vi "WaitBusy1212(Host).vi"(2 "error in":errorcluster, 3 "FPGA VI Reference In":refnum<k20>) -> (0 "error out":errorcluster, 1 "FPGA VI Reference Out":refnum<k20>)   [LabVIEW 2018]
uses:
  <vilib>/Utility/error.llb/Error Cluster From Error Code.vi
  <vilib>/rvi/errors/niLvFpgaAdjustHostInterfaceError.vi
  <vilib>/rvi/interface/nirviReadWriteControl/nirviReadWriteControl.xnode
  NiFpgaLv.dll
  <vilib>/rvi/interface/Simulation/niFpgaSimulationCallBeginRW.vi
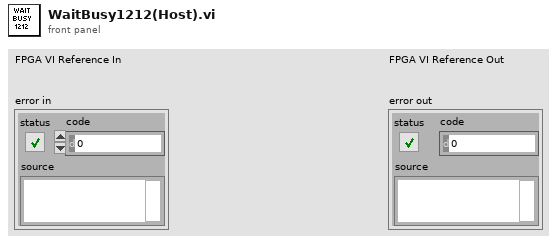
[diagram p1: front panel]
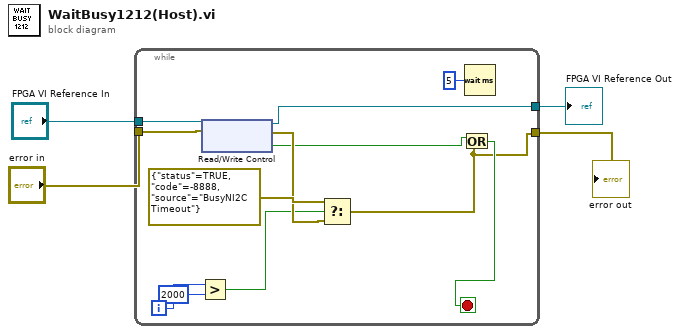
[diagram p0: block diagram]
diagram:
  n1 = while {
    tunnel: "FPGA VI Reference In" -> [w16]
    tunnel: "error in" -> [w15]
    tunnel: [w14] -> w2
    tunnel: [w6] -> w1
    i -> [w11]
    stop <- w7 stop-if-true
    n2 = Greater?(x=w11, y=2000) -> (0:w9:bool)
    n3 = xnode "Read/Write Control"("FPGA VI Reference In"=w16, "error in"=w15) -> ("FPGA VI Reference Out"=w14:refnum<k20>, "error out"=w12:errorcluster, "busy_ni2c"=w8:bool)
    n4 = Select(t=errorcluster {"status"=TRUE, "code"=-8888, "source"="BusyNI2C Timeout"} ("error out"), s=w9, f=w12) -> (s? t:f=w6:errorcluster)
    n5 = Or(x=w8, y=w6) -> (x .or. y?=w7:bool)
    n6 = Wait (ms)(milliseconds to wait=u32 5) -> ()  [unwired: 1 out]
  }
  "FPGA VI Reference Out" <- w2
  "error out" <- w1
